vi "Get Scenario Paths.vi"(8 "error in (no error)":errorcluster, 11 "Section Ref in":T1 format="%.0x") -> (0 "error out":errorcluster, 1 "Scenario Paths (path)":path[](array[path]), 2 "Scenario Paths (str)":string[](array[string]), 3 "Section Ref out":T1 format="%.0x")   [LabVIEW 2018, in "Vires VTD System Explorer.lvlib"]
uses:
  Vires VTD System Explorer.lvlib
  <vilib>/NI Veristand/Custom Device API/Custom Device Item Ref.ctl
  Shared/Constants.vi
  <vilib>/NI Veristand/Custom Device Tools/Custom Device Utility Library/NI VeriStand - Search for Item by GUID.vi
  <vilib>/NI Veristand/Custom Device API/Get Item Property (String Array).vi
  Shared/Vires VTD Shared.lvlib
  <vilib>/NI Veristand/Custom Device API/Custom Device API.lvlib
  <vilib>/NI Veristand/Custom Device Tools/Custom Device Utility Library/Custom Device Utility Library.lvlib
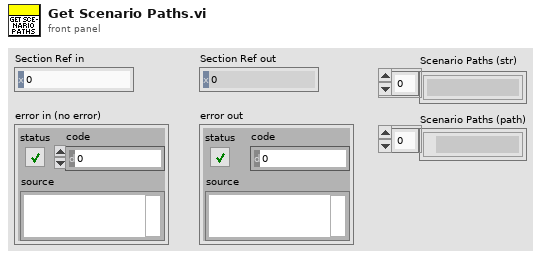
[diagram p1: front panel]
types:
  T1 = typedef "Custom Device API.lvlib/Custom Device Item Ref.ctl" = u64
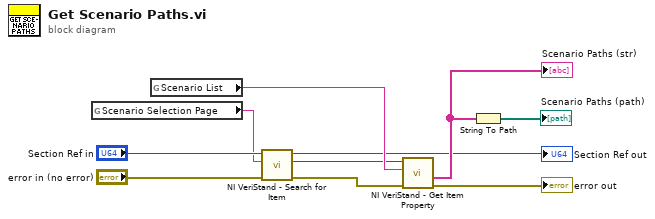
[diagram p0: block diagram]
diagram:
  n1 = global read "Constants.vi" "Scenario Selection Page"() -> (w8:string)
  n2 = global read "Constants.vi" "Scenario List"() -> (w7:string)
  n3 = call-poly <vilib>:"NI VeriStand - Search for Item.vi"("error in"="error in (no error)", "Item GUID"=w8, "Section Ref in"="Section Ref in") -> ("error out"=w6:errorcluster, "Item Ref"=w2:T1, "Section Ref out"=→"Section Ref out":T1)  [unwired: 5 in, 1 out]
  n4 = call-poly <vilib>:"NI VeriStand - Get Item Property.vi"("error in (no error)"=w6, "Property Name"=w7, "Item Ref in"=w2) -> ("error out"=→"error out":errorcluster, "Value"=w4:string[])  [unwired: 5 in, 2 out]
  "Scenario Paths (str)" <- w4
  n5 = String To Path(string=w4) -> (path=→"Scenario Paths (path)":path[])
